vi "drawradar_addTarget.vi"() -> ()   [LabVIEW 2014]
panel:
  in  "speed 3":u32(slide)=10 scale=100.0..1.0
  in  "speed 2":u32(slide)=10 scale=100.0..1.0
  in  "Style":T1(ring)
  in  "Width":u16=3
  out "th deg":i32
  in  "Direction":bool
  in  "speed":u32(slide)=10 scale=100.0..1.0
  in  "stop":bool
  in  "Color":u32(colorbox)=2621184
  out "picture":picture
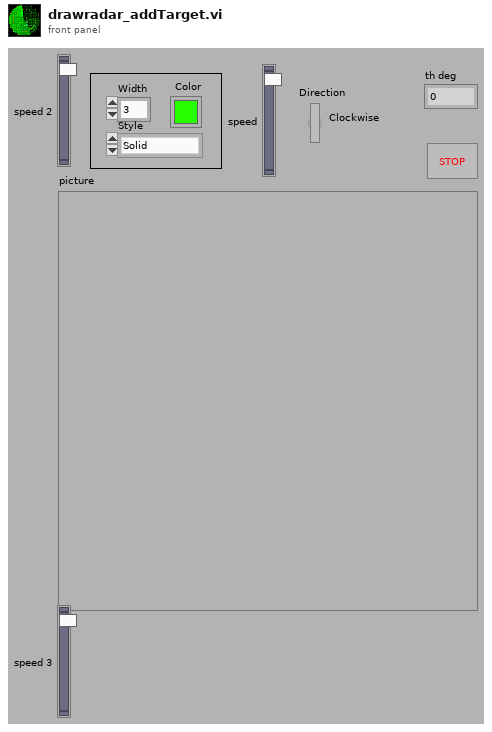
[diagram p1: front panel]
types:
  T1 = enum32{"Solid", "Dash", "Dot", "DashDot", "DashDotDot"}
  T2 = cluster{"Width":u16, "Style":enum32{"Solid", "Dash", "Dot", "DashDot", "DashDotDot"}}
  T3 = typedef "LVBoundsTypeDef.ctl" = cluster{"Width":u32, "Height":u32}
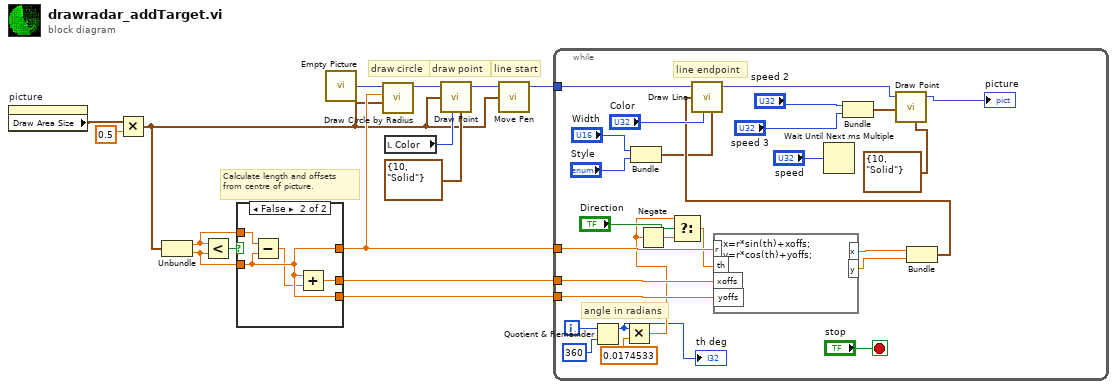
[diagram p0: block diagram]
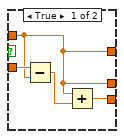
[diagram p2: hidden frame]
diagram:
  # "line start"
  # "draw point"
  # "draw circle"
  # "Calculate length and offsets from centre of picture."
  n1 = property on="picture" class="Pict"() -> ("Draw Area Size"=w13:T3)  [unwired: 2 in, 2 out]
  n2 = Multiply(x=w13, y=sgl 0.5) -> (x*y=w1:cluster{"Width":sgl, "Height":sgl})
  n3 = Unbundle(w1) -> ("Width"=w11:sgl, "Height"=w10:sgl)
  n4 = Less?(x=w11, y=w10) -> (x < y?=w12:bool)
  n5 = case shown="False" w12 {
    tunnel: [w17 w21] -> w6
    tunnel: w11 -> [w17 w23]
    tunnel: w10 -> [w18 w21]
    tunnel: [w17 w22] -> w9
    tunnel: [w19 w21] -> w8
    frame True {
      n6 = Subtract(x=w18, y=w17) -> (x-y=w16:sgl)
      n7 = Add(x=w17, y=w16) -> (x+y=w19:sgl)
    }
    frame False {
      n8 = Subtract(x=w23, y=w21) -> (x-y=w20:sgl)
      n9 = Add(x=w21, y=w20) -> (x+y=w22:sgl)
    }
  }
  n10 = call "Empty Picture"() -> ("empty picture"=w7:picture)
  n11 = call <vilib>:"Draw Circle by Radius.vi"("pixel center"=w1, "radius"=w6, "picture"=w7) -> ("new picture"=w5:picture)  [unwired: 5 in, 3 out]
  n12 = local read "Color"() -> (w3:u32)
  n13 = call <vilib>:"Draw Point.vi"("picture"=w5, "point(x,y)"=w1, "color(black)"=w3, "pen"=T2 {"Width"=10, "Style"=enum."Solid"}) -> ("new picture"=w4:picture)  [unwired: 5 out]
  n14 = call <vilib>:"Move Pen.vi"("new position"=w1, "picture"=w4) -> ("new picture"=w15:picture)  [unwired: 2 in, 1 out]
  n15 = while {
    tunnel: w15 -> [w50]
    tunnel: w6 -> [w40]
    tunnel: w9 -> [w39]
    tunnel: w8 -> [w38]
    i -> [w46]
    stop <- "stop" stop-if-true
    # "line endpoint"
    # "angle in radians"
    n16 = Quotient & Remainder(x=w46, y=360) -> (x-y*floor(x/y)=w33:i32)  [unwired: 1 out]
    "th deg" <- w33
    n17 = Multiply(x=w33, y=0.0174533 ("input variable")) -> (x*y=w35:dbl)
    n18 = Bundle("Width"="Width", "Style"="Style") -> (w30:T2)  [unwired: 1 out]
    n19 = Negate(x=w35) -> (-x=w34:dbl)
    n20 = Select(t=w35, s="Direction", f=w34) -> (s? t:f=w36:dbl)
    n21 = formula code="x=r*sin(th)+xoffs;\ny=r*cos(th)+yoffs;"("r"=w40, "th"=w36, "xoffs"=w39, "yoffs"=w38) -> ("x"=w44:dbl, "y"=w43:dbl)
    n22 = Wait Until Next ms Multiple(millisecond multiple="speed") -> ()  [unwired: 1 out]
    n23 = Bundle("speed 2"="speed 2", "speed 3"="speed 3") -> (w27:cluster{"speed 2":u32, "speed 3":u32})  [unwired: 1 out]
    n24 = Bundle("x"=w44, "y"=w43) -> (w42:cluster{"x":dbl, "y":dbl})  [unwired: 1 out]
    n25 = call <vilib>:"Draw Line.vi"("picture"=w50, "end point"=w42, "color(black)"="Color", "pen"=w30) -> ("new picture"=w29:picture)  [unwired: 1 in, 4 out]
    n26 = call <vilib>:"Draw Point.vi"("picture"=w29, "point(x,y)"=w27, "pen"=T2 {"Width"=10, "Style"=enum."Solid"}) -> ("new picture"=→"picture":picture)  [unwired: 6 in]
  }
